vi "Initialize Scalar Datatype Classes.vi"(8 "error in (no error)":errorcluster, 10 "Register":T4={"Name"="", "Data Type"=enum."<Null>", "Default Value"=variant(dbl 0.0)} {"Data Type" format="%.0x"}, 11 "FPGA Ref":refnum<k20>) -> (0 "error out":errorcluster, 2 "Register":T1 {"Data Type" format="%.0x"}, 3 "FPGA Ref":refnum<k20>)   [LabVIEW 2016, in "FPGA Addon Engine.lvlib"]
uses:
  FPGA Addon Engine.lvlib
  FPGA-Resource-Manager-APIs/Source/Shared/Types/Register Information.ctl
  FPGA-Resource-Manager-APIs/Source/Shared/Types/Data Type.ctl
  Types/Register Settings.ctl
  FPGA-Resource-Manager-APIs/Source/Shared/Types/Scalar Type.ctl
  <vilib>/NI/LVFPGA Adv Session Resources/OpenByNameSubVI.vi
  <vilib>/Utility/error.llb/Error Cluster From Error Code.vi
  <vilib>/rvi/interface/common/dynamic/niFpgaEscapeDelimiterAndNull.vi
  <vilib>/NI/LVFPGA Adv Session Resources/OpenByName.xnode
  <vilib>/NI/LVFPGA Adv Session Resources/LVFPGAAdvSessionResources.lvlib
  FPGA-Resource-Manager-APIs/Source/Shared/FPGA RM Shared API.lvlib
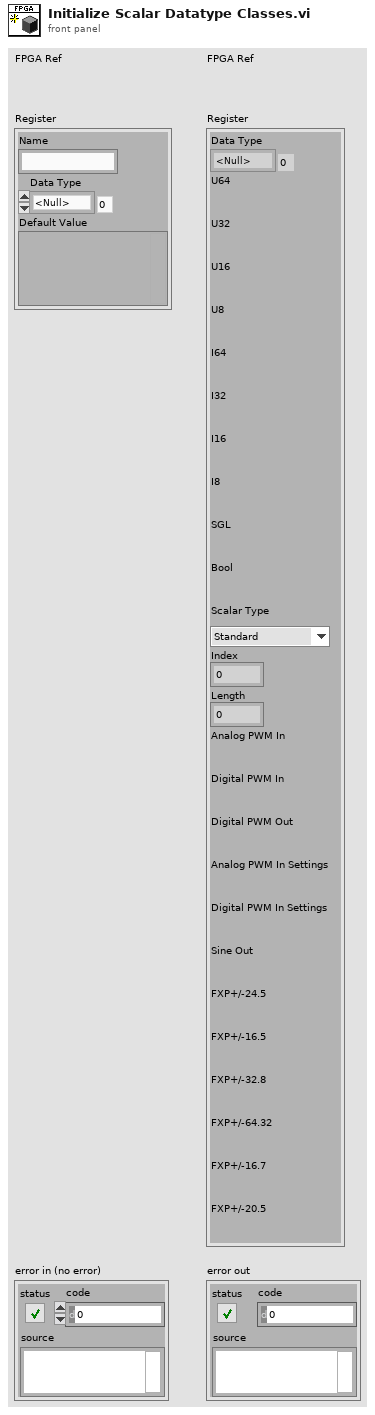
[diagram p1: front panel]
types:
  T1 = typedef "FPGA Addon Engine.lvlib/Register Settings.ctl" = cluster{"Data Type":T2, "U64":refnum<k20>, "U32":refnum<k20>, "U16":refnum<k20>, "U8":refnum<k20>, "I64":refnum<k20>, "I32":refnum<k20>, "I16":refnum<k20>, "I8":refnum<k20>, "SGL":refnum<k20>, "Bool":refnum<k20>, "Scalar Type":T3, "Index":i32, "Length":i32, "Analog PWM In":refnum<k20>, "Digital PWM In":refnum<k20>, "Digital PWM Out":refnum<k20>, "Analog PWM In Settings":refnum<k20>, "Digital PWM In Settings":refnum<k20>, "Sine Out":refnum<k20>, "FXP+/-24.5":refnum<k20>, "FXP+/-16.5":refnum<k20>, "FXP+/-32.8":refnum<k20>, "FXP+/-64.32":refnum<k20>, "FXP+/-16.7":refnum<k20>, "FXP+/-20.5":refnum<k20>}
  T2 = typedef "FPGA RM Shared API.lvlib/Data Type.ctl" = enum8{"<Null>", "I8", "I16", "I32", "I64", "U8", "U16", "U32", "U64", "SGL", "Boolean", "Analog PWM In Settings", "Analog PWM In", "Digital PWM In Settings", "Digital PWM In", "Digital PWM Out", "Sine Out", "FXP+/-24.5", "FXP+/-16.5", "FXP+/-32.8", "FXP+/-64.32", "FXP+/-16.7", "FXP+/-20.5"}
  T3 = typedef "FPGA RM Shared API.lvlib/Scalar Type.ctl" = enum16{"Standard", "Bitpacked"}
  T4 = typedef "FPGA RM Shared API.lvlib/Register Information.ctl" = cluster{"Name":string, "Data Type":T2, "Default Value":variant}
  T5 = cluster{"Name":string, "Depth":u32, "Write? (Deprecated:Use Implementation)":bool, "Physical Channel":u32, "Base Address":u32, "Data Width":u32, "Data Type":enum32{"Boolean", "I8", "I16", "I32", "I64", "U8", "U16", "U32", "U64", "FXP", "CustomControl", "SGL"}, "FXP Properties":variant, "Write Window Address":u32, "Implementation":enum16{"niFpgaTargetToHost", "niFpgaHostToTarget", "niFpgaPeerToPeerWriter", "niFpgaPeerToPeerReader", "niCoreTargetToHost", "niCoreHostToTarget"}, "Control Set":u32}[]
  T6 = cluster{"Name":string, "type":variant, "indicator?":bool}[]
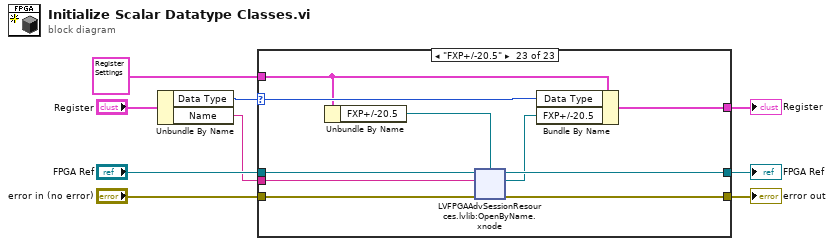
[diagram p0: block diagram]
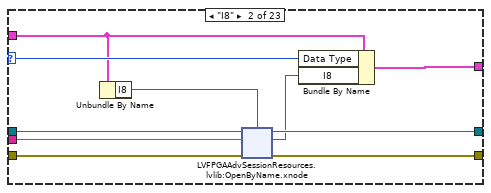
[diagram p3: hidden frame]
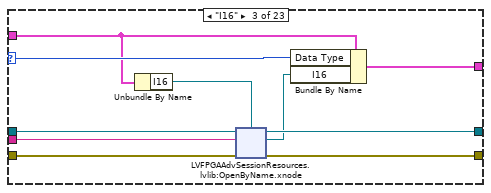
[diagram p4: hidden frame]
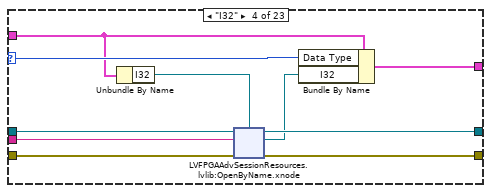
[diagram p5: hidden frame]
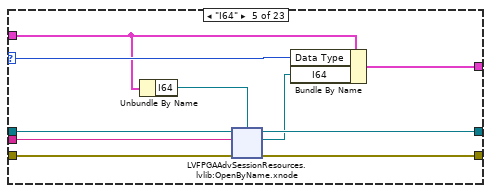
[diagram p6: hidden frame]
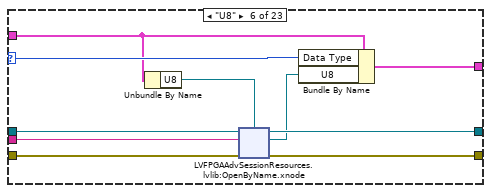
[diagram p7: hidden frame]
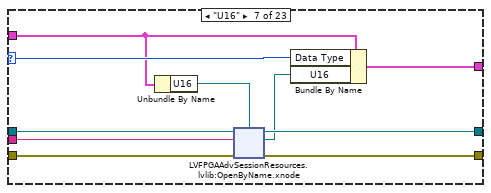
[diagram p8: hidden frame]
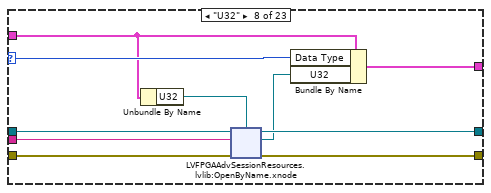
[diagram p9: hidden frame]
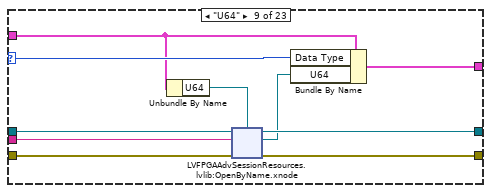
[diagram p10: hidden frame]
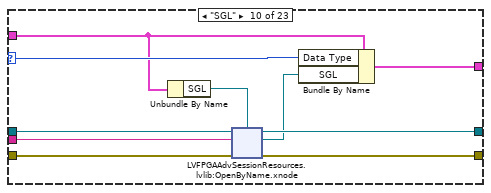
[diagram p11: hidden frame]
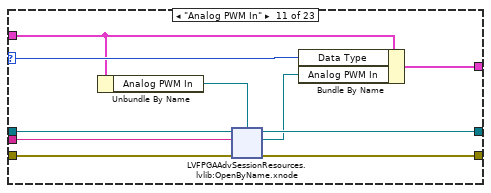
[diagram p12: hidden frame]
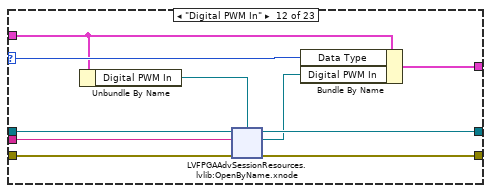
[diagram p13: hidden frame]
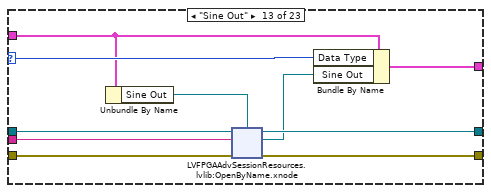
[diagram p14: hidden frame]
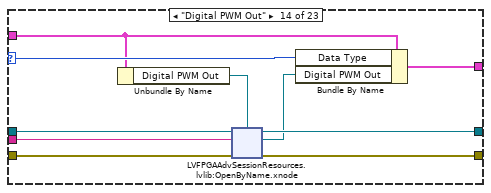
[diagram p15: hidden frame]
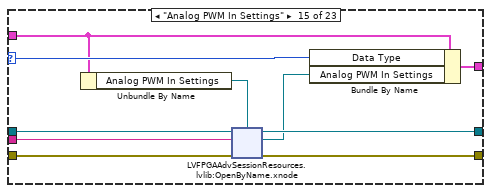
[diagram p16: hidden frame]
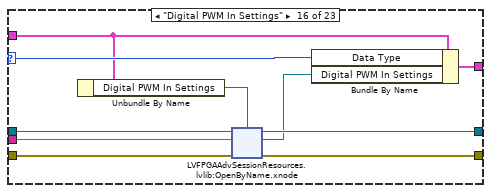
[diagram p17: hidden frame]
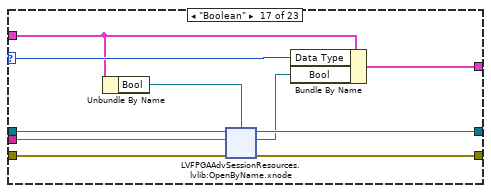
[diagram p18: hidden frame]
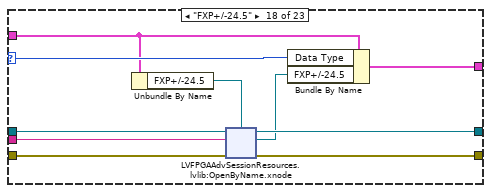
[diagram p19: hidden frame]
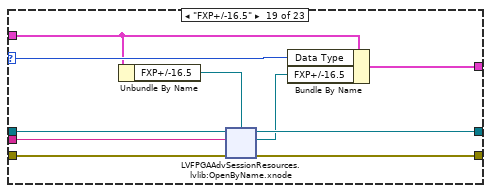
[diagram p20: hidden frame]
diagram:
  n1 = Unbundle By Name("Register") -> ("Data Type"=w2:T2, "Name"=w1:string)
  n2 = case shown="\"FXP+/-20.5\"" w2 {
    selector: w2 -> [_ w19 w42 w65 w88 w111 w134 w157 w180 w203 w226 w249 w272 w295 w318 w341 w363 w386 w409 w432 w455 w478 w501]
    tunnel: "FPGA Ref" -> [w12 w22 w45 w68 w91 w114 w137 w160 w183 w206 w229 w252 w275 w298 w321 w344 w367 w390 w413 w436 w459 w482 w505]
    tunnel: [w12 w20 w43 w66 w89 w112 w135 w158 w182 w204 w227 w250 w273 w296 w319 w342 w365 w388 w411 w434 w457 w480 w503] -> w9
    tunnel: w1 -> [_ w21 w44 w67 w90 w113 w136 w159 w181 w205 w228 w251 w274 w297 w320 w343 w366 w389 w412 w435 w458 w481 w504]
    tunnel: T1 {"Data Type"=enum."<Null>", "U64"=refnum, "U32"=refnum, "U16"=refnum, "U8"=refnum, "I64"=refnum, "I32"=refnum, "I16"=refnum, "I8"=refnum, "SGL"=refnum, "Bool"=refnum, "Scalar Type"=enum."Standard", "Index"=0, "Length"=0, "Analog PWM In"=refnum, "Digital PWM In"=refnum, "Digital PWM Out"=refnum, "Analog PWM In Settings"=refnum, "Digital PWM In Settings"=refnum, "Sine Out"=refnum, "FXP+/-24.5"=refnum, "FXP+/-16.5"=refnum, "FXP+/-32.8"=refnum, "FXP+/-64.32"=refnum, "FXP+/-16.7"=refnum, "FXP+/-20.5"=refnum} ("Cluster") -> [w11 w14 w37 w60 w83 w106 w129 w152 w175 w198 w221 w244 w267 w290 w314 w336 w359 w382 w405 w428 w451 w474 w497]
    tunnel: [w11 w17 w40 w63 w86 w109 w132 w155 w179 w201 w224 w247 w270 w293 w317 w339 w362 w385 w408 w431 w454 w477 w500] -> w4
    tunnel: "error in (no error)" -> [w10 w16 w39 w62 w85 w108 w130 w154 w176 w200 w223 w246 w269 w292 w316 w338 w361 w384 w407 w430 w453 w476 w499]
    tunnel: [w10 w15 w38 w61 w84 w107 w131 w153 w177 w199 w222 w245 w268 w291 w315 w337 w360 w383 w406 w429 w452 w475 w498] -> w8
    frame "<Null>", Default {
    }
    frame "I8" {
      n3 = Unbundle By Name(w14) -> ("I8"=w13:refnum<k20>)
      n4 = xnode "LVFPGAAdvSessionResources.lvlib:OpenByName.xnode"("FPGA VI Reference in"=w22, "Resource name in"=w21, "Single resource reference type in"=w13, "Error in"=w16) -> ("Single resource reference out"=w18:refnum<k20>, "Error out"=w15:errorcluster, "FPGA VI Reference out"=w20:refnum<k20>)
      n5 = Bundle By Name(cluster=w14, "Data Type"=w19, "I8"=w18) -> (w17:T1)
    }
    frame "I16" {
      n6 = Unbundle By Name(w37) -> ("I16"=w36:refnum<k20>)
      n7 = xnode "LVFPGAAdvSessionResources.lvlib:OpenByName.xnode"("FPGA VI Reference in"=w45, "Resource name in"=w44, "Single resource reference type in"=w36, "Error in"=w39) -> ("Single resource reference out"=w41:refnum<k20>, "Error out"=w38:errorcluster, "FPGA VI Reference out"=w43:refnum<k20>)
      n8 = Bundle By Name(cluster=w37, "Data Type"=w42, "I16"=w41) -> (w40:T1)
    }
    frame "I32" {
      n9 = Unbundle By Name(w60) -> ("I32"=w59:refnum<k20>)
      n10 = xnode "LVFPGAAdvSessionResources.lvlib:OpenByName.xnode"("FPGA VI Reference in"=w68, "Resource name in"=w67, "Single resource reference type in"=w59, "Error in"=w62) -> ("Single resource reference out"=w64:refnum<k20>, "Error out"=w61:errorcluster, "FPGA VI Reference out"=w66:refnum<k20>)
      n11 = Bundle By Name(cluster=w60, "Data Type"=w65, "I32"=w64) -> (w63:T1)
    }
    frame "I64" {
      n12 = Unbundle By Name(w83) -> ("I64"=w82:refnum<k20>)
      n13 = xnode "LVFPGAAdvSessionResources.lvlib:OpenByName.xnode"("FPGA VI Reference in"=w91, "Resource name in"=w90, "Single resource reference type in"=w82, "Error in"=w85) -> ("Single resource reference out"=w87:refnum<k20>, "Error out"=w84:errorcluster, "FPGA VI Reference out"=w89:refnum<k20>)
      n14 = Bundle By Name(cluster=w83, "Data Type"=w88, "I64"=w87) -> (w86:T1)
    }
    frame "U8" {
      n15 = Unbundle By Name(w106) -> ("U8"=w105:refnum<k20>)
      n16 = xnode "LVFPGAAdvSessionResources.lvlib:OpenByName.xnode"("FPGA VI Reference in"=w114, "Resource name in"=w113, "Single resource reference type in"=w105, "Error in"=w108) -> ("Single resource reference out"=w110:refnum<k20>, "Error out"=w107:errorcluster, "FPGA VI Reference out"=w112:refnum<k20>)
      n17 = Bundle By Name(cluster=w106, "Data Type"=w111, "U8"=w110) -> (w109:T1)
    }
    frame "U16" {
      n18 = Unbundle By Name(w129) -> ("U16"=w128:refnum<k20>)
      n19 = xnode "LVFPGAAdvSessionResources.lvlib:OpenByName.xnode"("FPGA VI Reference in"=w137, "Resource name in"=w136, "Single resource reference type in"=w128, "Error in"=w130) -> ("Single resource reference out"=w133:refnum<k20>, "Error out"=w131:errorcluster, "FPGA VI Reference out"=w135:refnum<k20>)
      n20 = Bundle By Name(cluster=w129, "Data Type"=w134, "U16"=w133) -> (w132:T1)
    }
    frame "U32" {
      n21 = Unbundle By Name(w152) -> ("U32"=w151:refnum<k20>)
      n22 = xnode "LVFPGAAdvSessionResources.lvlib:OpenByName.xnode"("FPGA VI Reference in"=w160, "Resource name in"=w159, "Single resource reference type in"=w151, "Error in"=w154) -> ("Single resource reference out"=w156:refnum<k20>, "Error out"=w153:errorcluster, "FPGA VI Reference out"=w158:refnum<k20>)
      n23 = Bundle By Name(cluster=w152, "Data Type"=w157, "U32"=w156) -> (w155:T1)
    }
    frame "U64" {
      n24 = Unbundle By Name(w175) -> ("U64"=w174:refnum<k20>)
      n25 = xnode "LVFPGAAdvSessionResources.lvlib:OpenByName.xnode"("FPGA VI Reference in"=w183, "Resource name in"=w181, "Single resource reference type in"=w174, "Error in"=w176) -> ("Single resource reference out"=w178:refnum<k20>, "Error out"=w177:errorcluster, "FPGA VI Reference out"=w182:refnum<k20>)
      n26 = Bundle By Name(cluster=w175, "Data Type"=w180, "U64"=w178) -> (w179:T1)
    }
    frame "SGL" {
      n27 = Unbundle By Name(w198) -> ("SGL"=w197:refnum<k20>)
      n28 = xnode "LVFPGAAdvSessionResources.lvlib:OpenByName.xnode"("FPGA VI Reference in"=w206, "Resource name in"=w205, "Single resource reference type in"=w197, "Error in"=w200) -> ("Single resource reference out"=w202:refnum<k20>, "Error out"=w199:errorcluster, "FPGA VI Reference out"=w204:refnum<k20>)
      n29 = Bundle By Name(cluster=w198, "Data Type"=w203, "SGL"=w202) -> (w201:T1)
    }
    frame "Analog PWM In" {
      n30 = Unbundle By Name(w221) -> ("Analog PWM In"=w220:refnum<k20>)
      n31 = xnode "LVFPGAAdvSessionResources.lvlib:OpenByName.xnode"("FPGA VI Reference in"=w229, "Resource name in"=w228, "Single resource reference type in"=w220, "Error in"=w223) -> ("Single resource reference out"=w225:refnum<k20>, "Error out"=w222:errorcluster, "FPGA VI Reference out"=w227:refnum<k20>)
      n32 = Bundle By Name(cluster=w221, "Data Type"=w226, "Analog PWM In"=w225) -> (w224:T1)
    }
    frame "Digital PWM In" {
      n33 = Unbundle By Name(w244) -> ("Digital PWM In"=w243:refnum<k20>)
      n34 = xnode "LVFPGAAdvSessionResources.lvlib:OpenByName.xnode"("FPGA VI Reference in"=w252, "Resource name in"=w251, "Single resource reference type in"=w243, "Error in"=w246) -> ("Single resource reference out"=w248:refnum<k20>, "Error out"=w245:errorcluster, "FPGA VI Reference out"=w250:refnum<k20>)
      n35 = Bundle By Name(cluster=w244, "Data Type"=w249, "Digital PWM In"=w248) -> (w247:T1)
    }
    frame "Sine Out" {
      n36 = Unbundle By Name(w267) -> ("Sine Out"=w266:refnum<k20>)
      n37 = xnode "LVFPGAAdvSessionResources.lvlib:OpenByName.xnode"("FPGA VI Reference in"=w275, "Resource name in"=w274, "Single resource reference type in"=w266, "Error in"=w269) -> ("Single resource reference out"=w271:refnum<k20>, "Error out"=w268:errorcluster, "FPGA VI Reference out"=w273:refnum<k20>)
      n38 = Bundle By Name(cluster=w267, "Data Type"=w272, "Sine Out"=w271) -> (w270:T1)
    }
    frame "Digital PWM Out" {
      n39 = Unbundle By Name(w290) -> ("Digital PWM Out"=w289:refnum<k20>)
      n40 = xnode "LVFPGAAdvSessionResources.lvlib:OpenByName.xnode"("FPGA VI Reference in"=w298, "Resource name in"=w297, "Single resource reference type in"=w289, "Error in"=w292) -> ("Single resource reference out"=w294:refnum<k20>, "Error out"=w291:errorcluster, "FPGA VI Reference out"=w296:refnum<k20>)
      n41 = Bundle By Name(cluster=w290, "Data Type"=w295, "Digital PWM Out"=w294) -> (w293:T1)
    }
    frame "Analog PWM In Settings" {
      n42 = Unbundle By Name(w314) -> ("Analog PWM In Settings"=w313:refnum<k20>)
      n43 = xnode "LVFPGAAdvSessionResources.lvlib:OpenByName.xnode"("FPGA VI Reference in"=w321, "Resource name in"=w320, "Single resource reference type in"=w313, "Error in"=w316) -> ("Single resource reference out"=w312:refnum<k20>, "Error out"=w315:errorcluster, "FPGA VI Reference out"=w319:refnum<k20>)
      n44 = Bundle By Name(cluster=w314, "Data Type"=w318, "Analog PWM In Settings"=w312) -> (w317:T1)
    }
    frame "Digital PWM In Settings" {
      n45 = Unbundle By Name(w336) -> ("Digital PWM In Settings"=w335:refnum<k20>)
      n46 = xnode "LVFPGAAdvSessionResources.lvlib:OpenByName.xnode"("FPGA VI Reference in"=w344, "Resource name in"=w343, "Single resource reference type in"=w335, "Error in"=w338) -> ("Single resource reference out"=w340:refnum<k20>, "Error out"=w337:errorcluster, "FPGA VI Reference out"=w342:refnum<k20>)
      n47 = Bundle By Name(cluster=w336, "Data Type"=w341, "Digital PWM In Settings"=w340) -> (w339:T1)
    }
    frame "Boolean" {
      n48 = Unbundle By Name(w359) -> ("Bool"=w358:refnum<k20>)
      n49 = xnode "LVFPGAAdvSessionResources.lvlib:OpenByName.xnode"("FPGA VI Reference in"=w367, "Resource name in"=w366, "Single resource reference type in"=w358, "Error in"=w361) -> ("Single resource reference out"=w364:refnum<k20>, "Error out"=w360:errorcluster, "FPGA VI Reference out"=w365:refnum<k20>)
      n50 = Bundle By Name(cluster=w359, "Data Type"=w363, "Bool"=w364) -> (w362:T1)
    }
    frame "FXP+/-24.5" {
      n51 = Unbundle By Name(w382) -> ("FXP+/-24.5"=w381:refnum<k20>)
      n52 = xnode "LVFPGAAdvSessionResources.lvlib:OpenByName.xnode"("FPGA VI Reference in"=w390, "Resource name in"=w389, "Single resource reference type in"=w381, "Error in"=w384) -> ("Single resource reference out"=w387:refnum<k20>, "Error out"=w383:errorcluster, "FPGA VI Reference out"=w388:refnum<k20>)
      n53 = Bundle By Name(cluster=w382, "Data Type"=w386, "FXP+/-24.5"=w387) -> (w385:T1)
    }
    frame "FXP+/-16.5" {
      n54 = Unbundle By Name(w405) -> ("FXP+/-16.5"=w404:refnum<k20>)
      n55 = xnode "LVFPGAAdvSessionResources.lvlib:OpenByName.xnode"("FPGA VI Reference in"=w413, "Resource name in"=w412, "Single resource reference type in"=w404, "Error in"=w407) -> ("Single resource reference out"=w410:refnum<k20>, "Error out"=w406:errorcluster, "FPGA VI Reference out"=w411:refnum<k20>)
      n56 = Bundle By Name(cluster=w405, "Data Type"=w409, "FXP+/-16.5"=w410) -> (w408:T1)
    }
    frame "FXP+/-32.8" {
      n57 = Unbundle By Name(w428) -> ("FXP+/-32.8"=w427:refnum<k20>)
      n58 = xnode "LVFPGAAdvSessionResources.lvlib:OpenByName.xnode"("FPGA VI Reference in"=w436, "Resource name in"=w435, "Single resource reference type in"=w427, "Error in"=w430) -> ("Single resource reference out"=w433:refnum<k20>, "Error out"=w429:errorcluster, "FPGA VI Reference out"=w434:refnum<k20>)
      n59 = Bundle By Name(cluster=w428, "Data Type"=w432, "FXP+/-32.8"=w433) -> (w431:T1)
    }
    frame "FXP+/-64.32" {
      n60 = Unbundle By Name(w451) -> ("FXP+/-64.32"=w450:refnum<k20>)
      n61 = xnode "LVFPGAAdvSessionResources.lvlib:OpenByName.xnode"("FPGA VI Reference in"=w459, "Resource name in"=w458, "Single resource reference type in"=w450, "Error in"=w453) -> ("Single resource reference out"=w456:refnum<k20>, "Error out"=w452:errorcluster, "FPGA VI Reference out"=w457:refnum<k20>)
      n62 = Bundle By Name(cluster=w451, "Data Type"=w455, "FXP+/-64.32"=w456) -> (w454:T1)
    }
    frame "FXP+/-16.7" {
      n63 = Unbundle By Name(w474) -> ("FXP+/-16.7"=w473:refnum<k20>)
      n64 = xnode "LVFPGAAdvSessionResources.lvlib:OpenByName.xnode"("FPGA VI Reference in"=w482, "Resource name in"=w481, "Single resource reference type in"=w473, "Error in"=w476) -> ("Single resource reference out"=w479:refnum<k20>, "Error out"=w475:errorcluster, "FPGA VI Reference out"=w480:refnum<k20>)
      n65 = Bundle By Name(cluster=w474, "Data Type"=w478, "FXP+/-16.7"=w479) -> (w477:T1)
    }
    frame "FXP+/-20.5" {
      n66 = Unbundle By Name(w497) -> ("FXP+/-20.5"=w496:refnum<k20>)
      n67 = xnode "LVFPGAAdvSessionResources.lvlib:OpenByName.xnode"("FPGA VI Reference in"=w505, "Resource name in"=w504, "Single resource reference type in"=w496, "Error in"=w499) -> ("Single resource reference out"=w502:refnum<k20>, "Error out"=w498:errorcluster, "FPGA VI Reference out"=w503:refnum<k20>)
      n68 = Bundle By Name(cluster=w497, "Data Type"=w501, "FXP+/-20.5"=w502) -> (w500:T1)
    }
  }
  "FPGA Ref" <- w9
  "error out" <- w8
  "Register" <- w4
